vi "Check pedal.vi"(7 "Micron config":T3, 8 "Pedal selector":T2[](array[typedef]), 10 "Mode controls":T1) -> (2 "New mode controls":T1)   [LabVIEW 2014]
uses:
  initialization/micron_config.ctl
  manipulator/squiggle/Host/i2c_interface.ctl
  manipulator/squiggle/Host/fpga_reference.ctl
  Micron params.ctl
  stimulus.ctl
  injection_point.ctl
  filtering/goal_loop_parms.ctl
  mode_conrols.ctl
  manipulator_cal.ctl
  asap/labview/testing/probe_calibration.ctl
  host/network_params.ctl
  cancellation/sq_control_params.ctl
  cancellation/decoupled_gain.ctl
  cancellation/estimation_controls.ctl
  control_selector.ctl
  <vilib>/DAQmx/read.llb/DAQmx Read (Digital 1D Bool 1Chan 1Samp).vi
panel:
  out "Last state":bool[](array[boolean])
  # "Locals:"
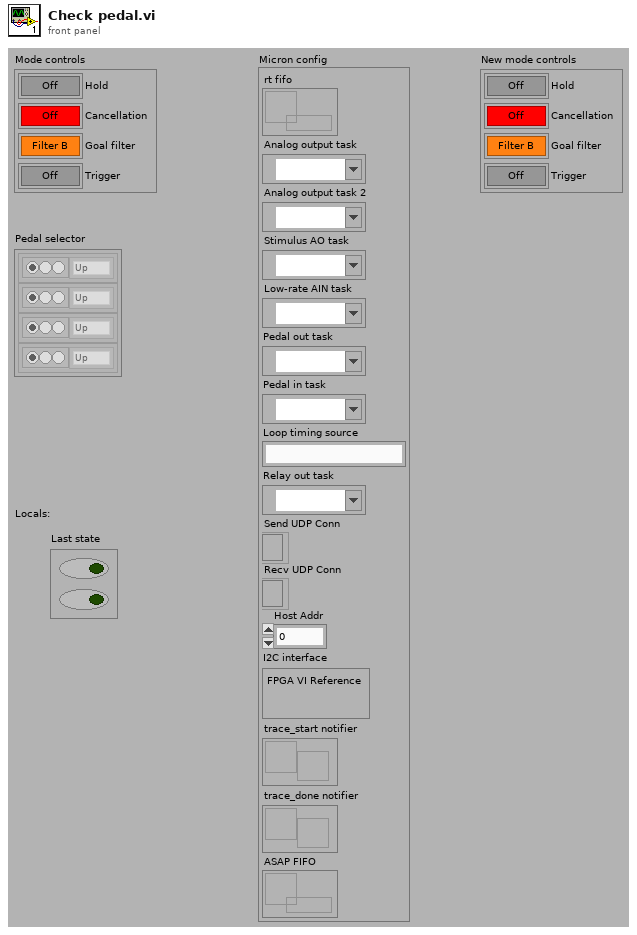
[diagram p1: front panel]
types:
  T1 = typedef "mode_conrols.ctl" = cluster{"Hold":bool, "Cancellation":bool, "Goal filter":bool, "Trigger":bool}
  T2 = typedef "control_selector.ctl" = cluster{"Selection":enum32{"No Selection", "Left", "Middle", "Right"}, "Mode":enum16{"Up", "Down", "Toggle", "Pulse", "Always", "Never"}}
  T3 = typedef "micron_config.ctl" = cluster{"rt fifo":refnum<k33>, "Analog output task":refnum<k21>, "Analog output task 2":refnum<k21>, "Stimulus AO task":refnum<k21>, "Low-rate AIN task":refnum<k21>, "Pedal out task":refnum<k21>, "Pedal in task":refnum<k21>, "Loop timing source":string, "Relay out task":refnum<k21>, "Send UDP Conn":refnum<k16>, "Recv UDP Conn":refnum<k16>, "Host Addr":u32, "I2C interface":T4, "trace_start notifier":refnum<notifier>, "trace_done notifier":refnum<notifier>, "ASAP FIFO":refnum<k33>}
  T4 = typedef "i2c_interface.ctl" = cluster{"FPGA VI Reference":T5}
  T5 = typedef "fpga_reference.ctl" = refnum<k20>
  T6 = enum32{"No Selection", "Left", "Middle", "Right"}
  T7 = enum16{"Up", "Down", "Toggle", "Pulse", "Always", "Never"}
  T8 = cluster{"[0]":bool, "[1]":bool, "[2]":bool, "[3]":bool}
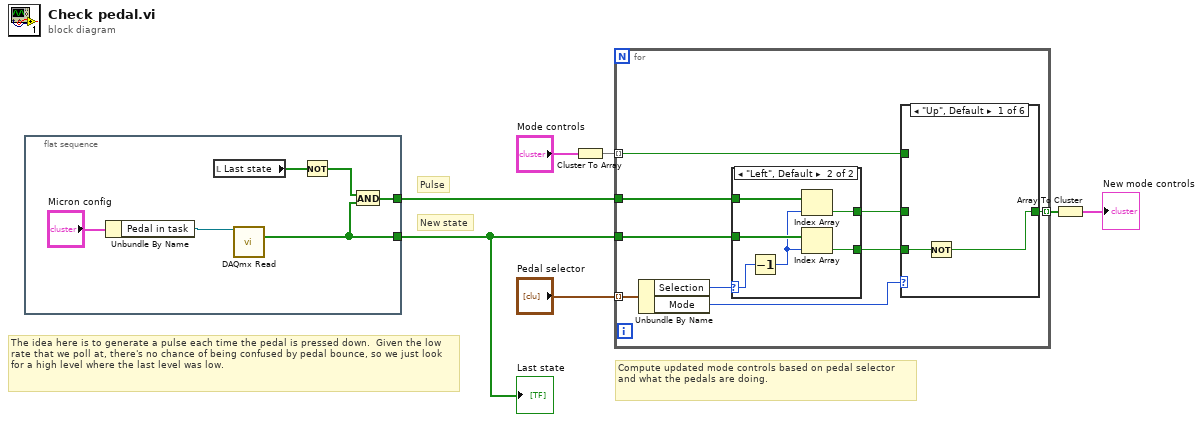
[diagram p0: block diagram]
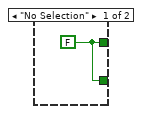
[diagram p2: hidden frame]
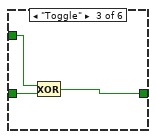
[diagram p4: hidden frame]
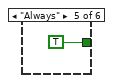
[diagram p6: hidden frame]
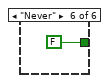
[diagram p7: hidden frame]
diagram:
  # "New state"
  # "Pulse"
  # "Compute updated mode controls based on pedal selector and what the pedals are doing."
  # "The idea here is to generate a pulse each time the pedal is pressed down.  Given the low rate that we poll at, there's no chance of being confused by pedal bounce, so we just look for a high level where the last level was low."
  n1 = flat-sequence {
    tunnel: [w11] -> w2
    tunnel: [w8] -> w1
    frame #0 {
      n2 = Unbundle By Name("Micron config") -> ("Pedal in task"=w13:refnum<k21>)
      n3 = local read "Last state"() -> (w9:bool[])
      n4 = call-poly <vilib>:"DAQmx Read.vi"("task/channels in"=w13) -> ("data"=w11:bool[])  [unwired: 2 in, 12 out]
      n5 = Not(x=w9) -> (.not. x?=w10:bool[])
      n6 = And(x=w10, y=w11) -> (x .and. y?=w8:bool[])
    }
  }
  n7 = Cluster To Array(cluster="Mode controls") -> (array=w6:bool[])
  n8 = for {
    tunnel: w6 -> [w18] mode=indexing
    tunnel: "Pedal selector" -> [w22] mode=indexing
    tunnel: w2 -> [w19]
    tunnel: w1 -> [w20]
    tunnel: [w15] -> w4 mode=indexing
    n9 = Unbundle By Name(w22) -> ("Selection"=w14:T6, "Mode"=w21:T7)
    n10 = case shown="\"Left\", Default" w14 {
      selector: w14 -> [_ w25]
      tunnel: w20 -> [_ w29]
      tunnel: w19 -> [_ w28]
      tunnel: [w23 w27] -> w17
      tunnel: [w23 w26] -> w16
      frame "No Selection" {
        w23 = FALSE ("Boolean")
      }
      frame "Left", Default {
        n11 = Decrement(x=w25) -> (x-1=w24:T6)
        n12 = Index Array(array=w29, index=w24) -> (element=w26:bool)
        n13 = Index Array(array=w28, index=w24) -> (element=w27:bool)
      }
    }
    n14 = case shown="\"Up\", Default" w21 {
      tunnel: [w31 w32 w33 w36 TRUE ("Boolean") FALSE ("Boolean")] -> w15
      tunnel: w18 -> [_ _ w34 _ _ _]
      tunnel: w17 -> [w30 w32 _ _ _ _]
      tunnel: w16 -> [_ _ w35 w36 _ _]
      frame "Up", Default {
        n15 = Not(x=w30) -> (.not. x?=w31:bool)
      }
      frame "Down" {
      }
      frame "Toggle" {
        n16 = Exclusive Or(1:w35, 2:w34) -> (0:w33:bool)
      }
      frame "Pulse" {
      }
      frame "Always" {
      }
      frame "Never" {
      }
    }
  }
  n17 = Array To Cluster(array=w4) -> (cluster=→"New mode controls":T8)
  "Last state" <- w2
